vi "Position to XML.vi"(8 "error in (no error)":errorcluster, 11 "focus in":refnum<class "focus.lvclass">) -> (0 "error out":errorcluster, 2 "XML string":string, 3 "focus out":refnum<class "focus.lvclass">)   [LabVIEW 2012, in "focus.lvclass"]
uses:
  focus.lvclass
  focus.lvclass/focus.ctl
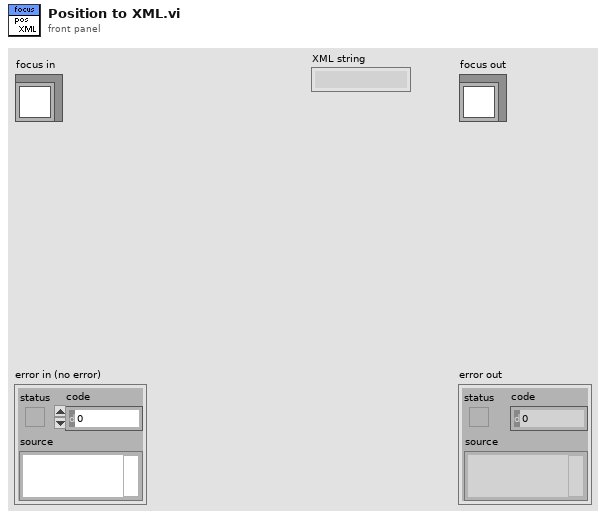
[diagram p1: front panel]
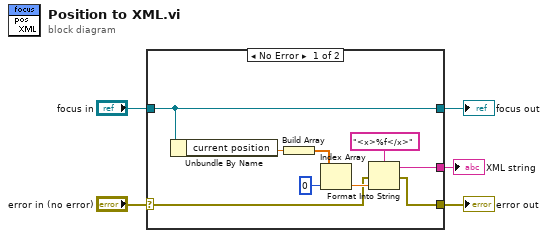
[diagram p0: block diagram]
diagram:
  n1 = case shown="No Error" "error in (no error)" {
    selector: "error in (no error)" -> [w9 w16]
    tunnel: [w8 w16] -> w4
    tunnel: [w14 w15] -> w2
    tunnel: "focus in" -> [w14 w15]
    tunnel: [w7 _] -> w1
    frame No Error {
      n2 = Unbundle By Name(w14) -> ("current position"=w12:dbl)
      n3 = Build Array(w12) -> (w11:dbl[])
      n4 = Index Array(array=w11, index=0) -> (element=w10:dbl)
      n5 = Format Into String(format string="<x>%f</x>", error in=w9, w10) -> (resulting string=w7:string, error out=w8:errorcluster)  [unwired: 1 in]
    }
    frame Error {
    }
  }
  "error out" <- w4
  "focus out" <- w2
  "XML string" <- w1
